vi "LakeShore 340 Set Power.vi"(3 "Heater Power (W)":sgl, 4 "Loop":u16(ring) items=["Loop 1", "Loop 2"], 5 "Lakeshore GPIB Address":refnum<visa-resource-name>) -> (1 "dup VISA session":refnum<visa-resource-name>)   [LabVIEW 2020]
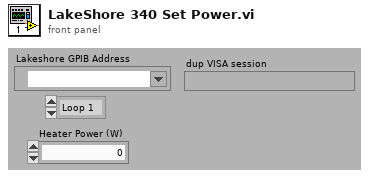
[diagram p1: front panel]
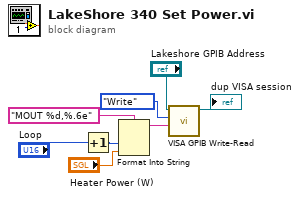
[diagram p0: block diagram]
diagram:
  n1 = Increment(x="Loop") -> (x+1=w1:u16)
  n2 = Format Into String(format string="MOUT %d,%.6e" ("initial string"), w1, "Heater Power (W)") -> (resulting string=w6:string)  [unwired: 2 in, 1 out]
  n3 = call "VISA GPIB Write-Read.vi"("Command"=w6, "Action"=enum16{"Write", "Read", "Write & Read"}."Write", "VISA resource name"="Lakeshore GPIB Address") -> ("dup VISA Session"=→"dup VISA session":refnum<visa-resource-name>)  [unwired: 5 in, 3 out]
